vi "Bind To Name.vi"(8 "error in (no error)":errorcluster, 10 "Type":refnum<class>, 11 "Known Types Binder in":refnum<class "Known Types Binder.lvclass">) -> (0 "error out":errorcluster, 2 "Type Name":string, 3 "Known Types Binder out":refnum<class "Known Types Binder.lvclass">)   [LabVIEW 2017, in "Known Types Binder.lvclass"]
doc: "Controls the binding of a type to a serialized object."
uses:
  Known Types Binder.lvclass
  Known Types Binder.lvclass/Known Types Binder.ctl
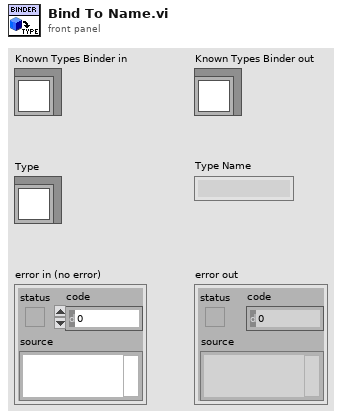
[diagram p1: front panel]
types:
  T1 = typedef "Known Types Binder.lvclass/Known Type.ctl" = cluster{"Name":string, "Type":refnum<class>}
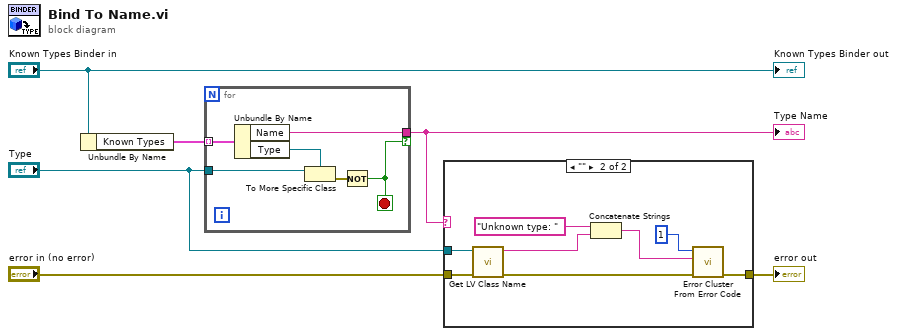
[diagram p0: block diagram]
diagram:
  n1 = Unbundle By Name("Known Types Binder in") -> ("Known Types"=w4:T1[])
  n2 = for {
    tunnel: w4 -> [w12] mode=indexing
    tunnel: "Type" -> [w10]
    tunnel: [w11] -> w1 if=w7
    stop <- w7 stop-if-true
    n3 = Unbundle By Name(w12) -> ("Name"=w11:string, "Type"=w9:refnum<class>)
    n4 = To More Specific Class(target class=w9, reference=w10) -> (error out=w8:errorcluster)  [unwired: 1 in, 1 out]
    n5 = Not(x=w8) -> (.not. x?=w7:bool)
  }
  "Type Name" <- w1
  n6 = case shown="\"\"" w1 {
    tunnel: "error in (no error)" -> [w13 w21]
    tunnel: [w13 w20] -> w3
    tunnel: "Type" -> [_ w17]
    frame Default {
    }
    frame "" {
      n7 = call <vilib>:"Get LV Class Name.vi"("error in (no error)"=w21, "object"=w17) -> ("error out"=w18:errorcluster, "class name"=w15:string)  [unwired: 8 in]
      n8 = Concatenate Strings("Unknown type: " ("string"), w15) -> (w14:string)
      n9 = call <vilib>:"Error Cluster From Error Code.vi"("error in (no error)"=w18, "error message (\"\")"=w14, "error code (0)"=1) -> ("error out"=w20:errorcluster)  [unwired: 6 in]
    }
  }
  "error out" <- w3
  "Known Types Binder out" <- "Known Types Binder in"
